vi "Abbreviate_Meas.vi"() -> (5 "Plug in titles":string[](array[string]), 7 "Plug in values":string[](array[string]))   [LabVIEW 2010]
uses:
  Globals/Meas_global.vi
panel:
  in  "Evaluation Time (s)":dbl=30.0
  in  "Theshold Concentration (ppm)":dbl=0.5 format="%_2g"
  # "You must have just these two indicators on the connector pane of the vi"
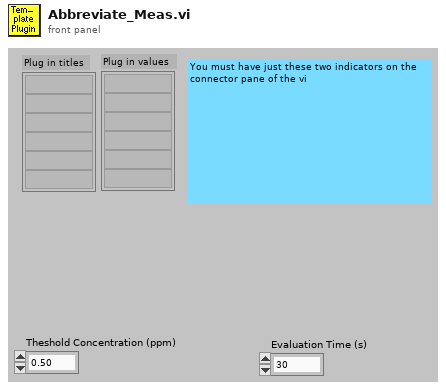
[diagram p1: front panel]
types:
  T1 = typedef "Post_Process.ctl" = enum16{"Take New Data", "Post Process Raw Data File"}
  T2 = typedef "Velocity_cluster.ctl" = cluster{"Name":string, "U":dbl, "u^2":dbl, "u^3/(u^2)^(1.5)":dbl, "u^4/(u^2)^2 -3":dbl, "% u'/U":dbl, "Mean % Err":dbl, "u^4":dbl}
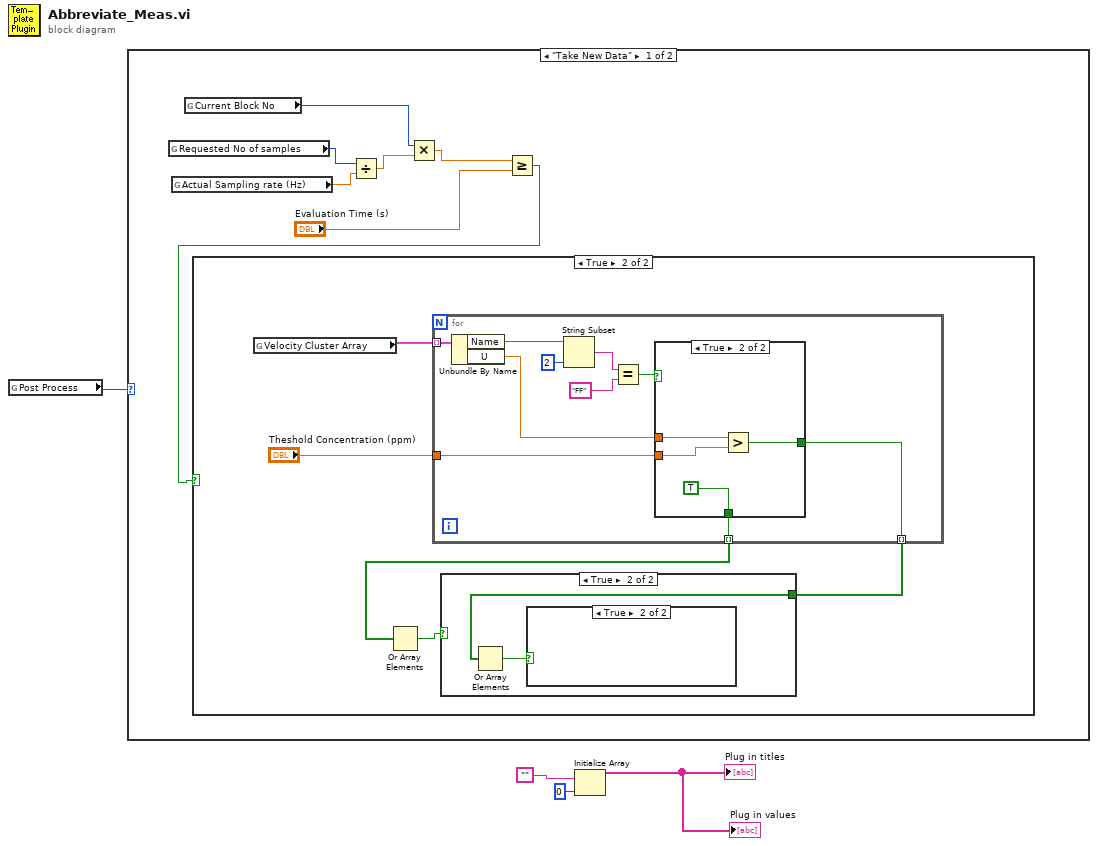
[diagram p0: block diagram]
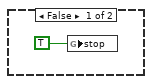
[diagram p4: hidden frame]
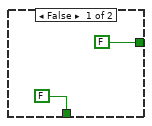
[diagram p5: hidden frame]
diagram:
  n1 = global read "Meas_global.vi" "Post Process"() -> (w4:T1)
  n2 = case shown="\"Take New Data\"" w4 {
    frame "Take New Data" {
      n3 = global read "Meas_global.vi" "Requested No of samples"() -> (w10:i32)
      n4 = global read "Meas_global.vi" "Actual Sampling rate (Hz)"() -> (w11:dbl)
      n5 = global read "Meas_global.vi" "Current Block No"() -> (w8:i32)
      n6 = Divide(x=w10, y=w11) -> (x/y=w9:dbl)
      n7 = Multiply(x=w8, y=w9) -> (x*y=w7:dbl)
      n8 = Greater Or Equal?(x=w7, y="Evaluation Time (s)") -> (x >= y?=w5:bool)
      n9 = case shown="True" w5 {
        frame False {
        }
        frame True {
          n10 = global read "Meas_global.vi" "Velocity Cluster Array"() -> (w16:T2[])
          n11 = for {
            tunnel: w16 -> [w29] mode=indexing
            tunnel: "Theshold Concentration (ppm)" -> [w22]
            tunnel: [w21] -> w14 mode=indexing
            tunnel: [w20] -> w13 mode=indexing
            n12 = Unbundle By Name(w29) -> ("Name"=w28:string, "U"=w23:dbl)
            n13 = String Subset(string=w28, length (rest)=2 ("length (rest)")) -> (substring=w26:string)  [unwired: 1 in]
            n14 = Equal?(x=w26, y="FF") -> (x = y?=w24:bool)
            n15 = case shown="True" w24 {
              tunnel: w23 -> [_ w35]
              tunnel: w22 -> [_ w34]
              tunnel: [FALSE w33] -> w21
              tunnel: [FALSE TRUE] -> w20
              frame False {
              }
              frame True {
                n16 = Greater?(x=w35, y=w34) -> (0:w33:bool)
              }
            }
          }
          n17 = Or Array Elements(Boolean array=w13) -> (logical OR=w12:bool)
          n18 = case shown="True" w12 {
            tunnel: w14 -> [_ w18]
            frame False {
            }
            frame True {
              n19 = Or Array Elements(Boolean array=w18) -> (logical OR=w17:bool)
              n20 = case shown="True" w17 {
                frame False {
                  n21 = global write "Meas_global.vi" "stop"(TRUE ("stop")) -> ()
                }
                frame True {
                }
              }
            }
          }
        }
      }
    }
    frame "Post Process Raw Data File" {
    }
  }
  n22 = Initialize Array("", 0) -> (→"Plug in values" →"Plug in titles":string[])
